vi "Parse Named Entry.vi"(7 "SpreadsheetDocument in":refnum<k24>, 8 "error in":errorcluster, 9 "Cells":variant, 10 "Named Range":string, 11 "<JSON>":string="{}") -> (0 "error out":errorcluster, 3 "<JSON> out":string)   [LabVIEW 2020, in "Configuration.lvlib" / "Config from EXCEL.lvclass"]
uses:
  Config from EXCEL.lvclass
  <vilib>/Peter/Open Xml/Source/DocumentFormat.OpenXml.dll
  <vilib>/JDP Science/JSONtext/LVClass Serializer/JSONtext LVClass Serializer.lvclass
  Config from EXCEL.lvclass/Config from EXCEL.ctl
  3d530874-43db-4d28-b45c-a44206ee6d76.vi
  <vilib>/JDP Science/JSONtext/JSONtext.lvlib
  <vilib>/Peter/Open Xml/Source/Open Xml.lvlib
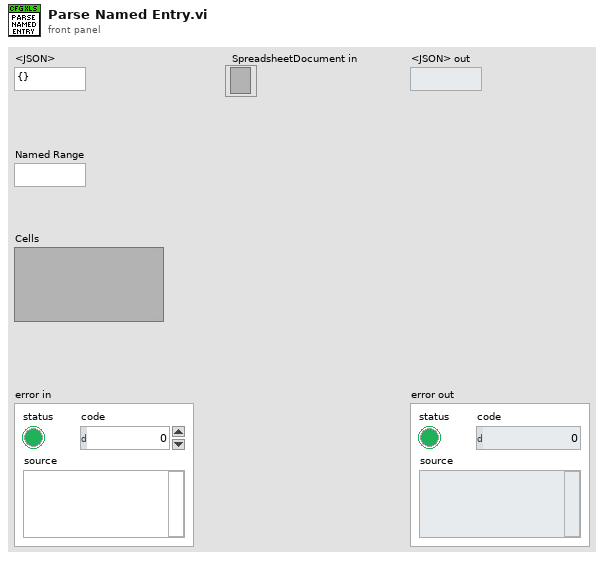
[diagram p1: front panel]
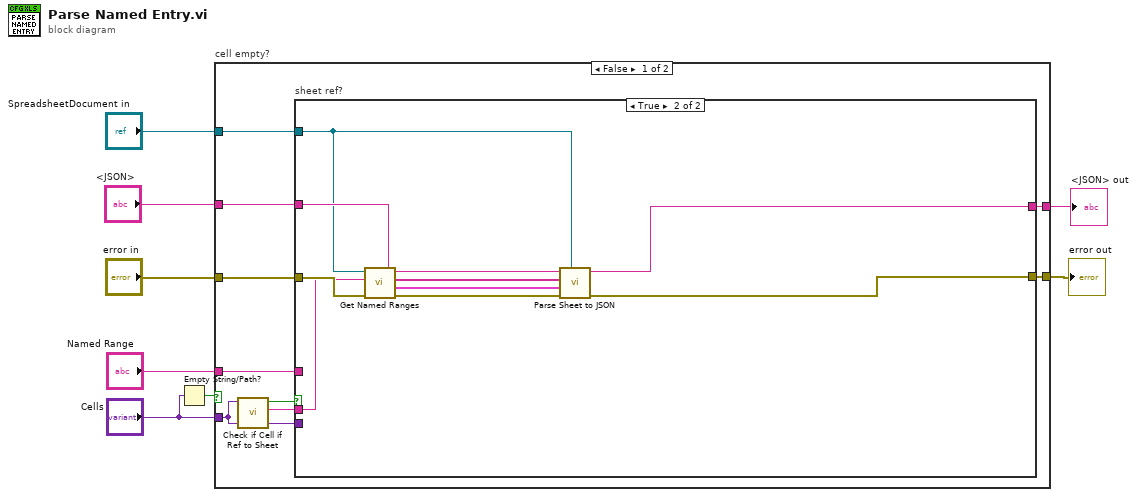
[diagram p0: block diagram]
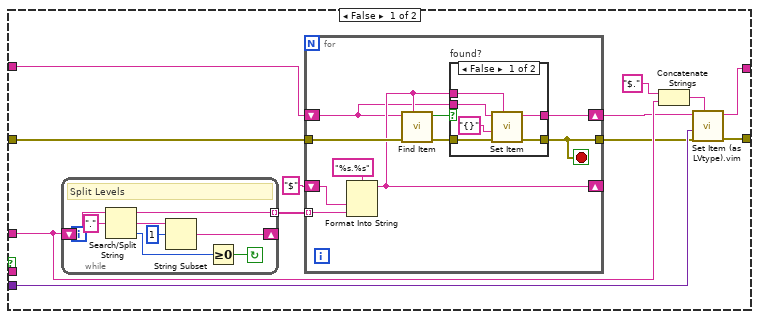
[diagram p2: hidden frame]
diagram:
  n1 = Empty String/Path?(string/path="Cells") -> (empty?=w2:bool)
  n2 = case "cell empty?" shown="False" w2 {
    tunnel: "error in" -> [w17 w66]
    tunnel: "SpreadsheetDocument in" -> [w16 _]
    tunnel: "Cells" -> [w13 _]
    tunnel: "<JSON>" -> [w12 w65]
    tunnel: "Named Range" -> [w11 _]
    tunnel: [w10 w66] -> w3
    tunnel: [w9 w65] -> w4
    frame False {
      n3 = call "Check if Cell if Ref to Sheet.vi"("Value"=w13) -> ("Sheet Name"=w15:string, "Sheet Ref"=w14:bool)  [unwired: 9 in]
      n4 = case "sheet ref?" shown="True" w14 {
        tunnel: w17 -> [w21 w64]
        tunnel: w16 -> [_ w56]
        tunnel: w15 -> [_ w63]
        tunnel: [w25 w61] -> w10
        tunnel: w13 -> [w27 _]
        tunnel: w12 -> [w18 w57]
        tunnel: w11 -> [w24 _]
        tunnel: [w26 w60] -> w9
        frame False {
          n5 = while {
            shift-right: [w50] -> _
            shift-left: w24 -> [w49]
            tunnel: [w48] -> w23 mode=indexing
            stop <- w51 continue-if-true
            # "Split Levels"
            n6 = Search/Split String(string=w49, search string/char (-)=".") -> (substring before match=w48:string, match + rest of string=w52:string, offset of match=w54:i32)  [unwired: 1 in]
            n7 = String Subset(string=w52, offset (0)=1) -> (substring=w50:string)  [unwired: 1 in]
            n8 = Greater Or Equal To 0?(x=w54) -> (x >= 0?=w51:bool)
          }
          n9 = for {
            tunnel: w23 -> [w37] mode=indexing
            shift-right: [w32] -> _
            shift-left: "$" -> [w38]
            tunnel: w21 -> [w35]
            tunnel: [w34] -> w20
            shift-right: [w31] -> w19
            shift-left: w18 -> [w30]
            stop <- w34 stop-if-true
            n10 = Format Into String(format string="%s.%s", w38, w37) -> (resulting string=w32:string)  [unwired: 2 in, 1 out]
            n11 = call <vilib>:"Find Item.vi"("$Path or Item Name"=w32, "error in (no error)"=w35, "JSON"=w30) -> ("error out"=w36:errorcluster, "Found"=w33:bool)  [unwired: 5 in, 2 out]
            n12 = case "found?" shown="False" w33 {
              tunnel: [w44 w46] -> w31
              tunnel: [w43 w47] -> w34
              tunnel: w36 -> [w42 w47]
              tunnel: w32 -> [w41 _]
              tunnel: w30 -> [w40 w46]
              frame False {
                n13 = call <vilib>:"Set Item.vi"("$Path or Item Name"=w41, "error in (no error)"=w42, "JSON to Insert"="{}", "JSON"=w40) -> ("error out"=w43:errorcluster, "<JSON>"=w44:string)  [unwired: 4 in, 1 out]
              }
              frame True {
              }
            }
          }
          n14 = Concatenate Strings("$." ("string"), w24) -> (w28:string)
          n15 = call "Set Item (as LVtype).vim"("$Path or Item Name"=w28, "error in (no error)"=w20, "Anything"=w27, "JSON"=w19) -> ("error out"=w25:errorcluster, "<JSON>"=w26:string)  [unwired: 4 in, 1 out]
        }
        frame True {
          n16 = call <vilib>:"Get Named Ranges.vi"("error in"=w64, "Sheet Name"=w63, "SpreadsheetDoc in"=w56) -> ("error out"=w62:errorcluster, "Cells"=w59:cluster{"Cells":variant[][]}[], "Range Names"=w58:string[])  [unwired: 5 in, 1 out]
          n17 = call "Parse Sheet to JSON.vi"("SpreadsheetDocument in"=w56, "error in"=w62, "Cells"=w59, "Named Ranges"=w58, "<JSON> in"=w57) -> ("error out"=w61:errorcluster, "<JSON> out"=w60:string)  [unwired: 5 in]
        }
      }
    }
    frame True {
    }
  }
  "error out" <- w3
  "<JSON> out" <- w4
